vi "Manual_Set_Temp_Value.vi"(11 "Output All":string) -> (3 "Manual Set Temp (C)":string)   [LabVIEW 2015]
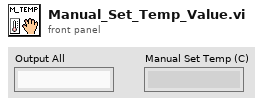
[diagram p1: front panel]
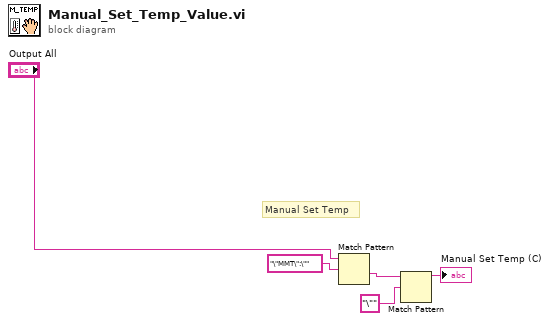
[diagram p0: block diagram]
diagram:
  # "Manual Set Temp"
  n1 = Match Pattern(string="Output All", regular expression="\"MMT\":\"") -> (after substring=w3:string)  [unwired: 1 in, 3 out]
  n2 = Match Pattern(string=w3, regular expression="\"") -> (before substring=→"Manual Set Temp (C)":string)  [unwired: 1 in, 3 out]
